vi "SP_OEE_2_test.vi"() -> ()   [LabVIEW 2017] (continued)
                      tunnel: [w10534] -> w10370
                      tunnel: [w10533] -> w10369
                      tunnel: [w10532] -> w10368
                      tunnel: [w10531] -> w10367
                      tunnel: [w10528] -> w10366
                      tunnel: [w10522] -> w10365
                      tunnel: [w10521] -> w10364
                      tunnel: [w10526] -> w10363
                      tunnel: [w10525] -> w10362
                      tunnel: [w10524] -> w10361
                      tunnel: w10374 -> [w10520]
                      tunnel: [w10520] -> w10360
                      tunnel: w10373 -> [w10517]
                      tunnel: [w10517] -> w10359
                      tunnel: [w10516] -> w10358
                      tunnel: w10372 -> [w10516]
                      tunnel: w10305 -> [w10515]
                      tunnel: [w10515] -> w10304
                      tunnel: w10299 -> [w10514]
                      tunnel: [w10514] -> w10298
                      tunnel: w10371 -> [w10559]
                      tunnel: w10370 -> [w10558]
                      tunnel: w10369 -> [w10557]
                      tunnel: w10368 -> [w10556]
                      tunnel: w10367 -> [w10555]
                      tunnel: w10366 -> [w10551]
                      tunnel: w10365 -> [w10554]
                      tunnel: w10364 -> [w10553]
                      tunnel: w10363 -> [w10550]
                      tunnel: w10362 -> [w10547]
                      tunnel: w10361 -> [w10546]
                      tunnel: [w10559] -> w10357
                      tunnel: [w10558] -> w10356
                      tunnel: [w10557] -> w10355
                      tunnel: [w10556] -> w10354
                      tunnel: [w10555] -> w10353
                      tunnel: [w10554] -> w10352
                      tunnel: [w10553] -> w10351
                      tunnel: [w10549] -> w10350
                      tunnel: [w10548] -> w10349
                      tunnel: [w10544] -> w10348
                      tunnel: [w10543] -> w10347
                      tunnel: [w10547] -> w10346
                      tunnel: [w10546] -> w10345
                      tunnel: w10360 -> [w10542]
                      tunnel: [w10542] -> w10344
                      tunnel: w10359 -> [w10539]
                      tunnel: [w10539] -> w10343
                      tunnel: [w10538] -> w10342
                      tunnel: w10358 -> [w10538]
                      tunnel: w10304 -> [w10537]
                      tunnel: [w10537] -> w10303
                      tunnel: w10298 -> [w10536]
                      tunnel: [w10536] -> w10297
                      tunnel: w10357 -> [w10585]
                      tunnel: w10356 -> [w10584]
                      tunnel: w10355 -> [w10583]
                      tunnel: w10354 -> [w10582]
                      tunnel: w10353 -> [w10581]
                      tunnel: w10352 -> [w10580]
                      tunnel: w10351 -> [w10579]
                      tunnel: w10350 -> [w10573]
                      tunnel: w10349 -> [w10575]
                      tunnel: w10348 -> [w10578]
                      tunnel: w10347 -> [w10577]
                      tunnel: w10346 -> [w10570]
                      tunnel: w10345 -> [w10571]
                      tunnel: [w10585] -> w10341
                      tunnel: [w10584] -> w10340
                      tunnel: [w10583] -> w10339
                      tunnel: [w10582] -> w10338
                      tunnel: [w10581] -> w10337
                      tunnel: [w10580] -> w10336
                      tunnel: [w10579] -> w10335
                      tunnel: [w10578] -> w10334
                      tunnel: [w10577] -> w10333
                      tunnel: [w10574] -> w10332
                      tunnel: [w10572] -> w10331
                      tunnel: [w10568] -> w10330
                      tunnel: [w10566] -> w10329
                      tunnel: w10344 -> [w10567]
                      tunnel: w10343 -> [w10563]
                      tunnel: [w10562] -> w10328
                      tunnel: w10342 -> [w10562]
                      tunnel: w10303 -> [w10561]
                      tunnel: w10297 -> [w10560]
                      tunnel: w10341 -> [w10612]
                      tunnel: w10340 -> [w10605]
                      tunnel: w10339 -> [w10596]
                      tunnel: w10338 -> [w10604]
                      tunnel: w10337 -> [w10594]
                      tunnel: w10336 -> [w10603]
                      tunnel: w10335 -> [w10592]
                      tunnel: w10334 -> [w10602]
                      tunnel: w10333 -> [w10590]
                      tunnel: w10332 -> [w10626]
                      tunnel: w10331 -> [w10625]
                      tunnel: w10330 -> [w10601]
                      tunnel: w10329 -> [w10588]
                      tunnel: [w10626] -> w10327
                      tunnel: [w10625] -> w10326
                      tunnel: [w10619] -> w10325
                      tunnel: [w10612] -> w10324
                      tunnel: [w10611] -> w10323
                      tunnel: [w10610] -> w10322
                      tunnel: [w10609] -> w10321
                      tunnel: [w10608] -> w10320
                      tunnel: [w10607] -> w10319
                      tunnel: [w10606] -> w10318
                      tunnel: [w10605] -> w10317
                      tunnel: [w10604] -> w10316
                      tunnel: [w10603] -> w10315
                      tunnel: [w10602] -> w10314
                      tunnel: [w10601] -> w10313
                      tunnel: [w10586] -> w10312
                      tunnel: w10328 -> [w10586]
                      tunnel: [w10646] -> w10288
                      tunnel: [w10632] -> w10286
                      tunnel: w10327 -> [w10633]
                      tunnel: w10326 -> [w10646]
                      tunnel: w10325 -> [w10631]
                      tunnel: w10324 -> [w10644]
                      tunnel: w10323 -> [w10642]
                      tunnel: w10322 -> [w10640]
                      tunnel: w10321 -> [w10638]
                      tunnel: w10320 -> [w10636]
                      tunnel: w10319 -> [w10634]
                      tunnel: w10318 -> [w10627]
                      tunnel: w10317 -> [w10643]
                      tunnel: w10316 -> [w10641]
                      tunnel: w10315 -> [w10639]
                      tunnel: w10314 -> [w10637]
                      tunnel: w10313 -> [w10635]
                      tunnel: w10312 -> [w10630]
                      tunnel: [w10627] -> w10296
                      frame #0 {
                        w10417 = "%Y-%m-%d" ("time format string (%c)")
                        n1887 = Decimal String To Number(string=w10404) -> (number=w10403:i32)  [unwired: 2 in, 1 out]
                        n1888 = property on="Table" class="Tbl (strict)"("Visible"=TRUE) -> ()  [unwired: 2 in, 2 out]
                        n1889 = Format Date/Time String(time format string (%c)=w10417, seconds (now)=w10409) -> (date/time string=w10418:string)  [unwired: 1 in]
                        n1890 = Format Date/Time String(time format string (%c)=w10417, seconds (now)=w10408) -> (date/time string=w10416:string)  [unwired: 1 in]
                        n1891 = Format Into String(format string="Where BREAKDOWN_DATE between '%s' and '%s' and  SHIFT_ID = '%d'  ", w10418, w10416, w10403) -> (resulting string=w10415:string)  [unwired: 2 in, 1 out]
                        n1892 = call <vilib>:"DB Tools Select Data.vi"("condition"=w10415, "error in (no error)"=w10424, "columns"=string[] ["BREAKDOWN_DATE"], "table"="STATION_1_LOG_HISTORY", "connection reference"=w10426) -> ("error out"=w10411:errorcluster, "data"=w10414:variant[][], "connection reference out"=w10425:T2)  [unwired: 1 in]
                        n1893 = property on="Table 2" class="Tbl (strict)"("Visible"=FALSE) -> ()  [unwired: 2 in, 2 out]
                        n1894 = xnode "Database Variant To Data"("database variant"=w10414, "error in (no error)"=w10411, "type"=string[][] [] ("Elements Found")) -> ("data"=w10412:string[][], "error out"=w10410:errorcluster)
                        n1895 = Index Array(array=w10412, index (col)=0 ("disabled index (col)")) -> (element=w10420:string[])  [unwired: 1 in]
                        n1896 = call "Search_1d_array_element.vi"("Count in"=string[] [] ("Elements Found"), "BD Date"=w10420, "Elements Found in"=string[] [] ("Elements Found")) -> ("Elements Found out"=w10406:string[])  [unwired: 4 in, 2 out]
                        n1897 = Build Array(w10406) -> (w10430:string[][])
                        n1898 = Transpose 2D Array(2D array=w10430) -> (transposed array=w10429:string[][])
                      }
                      frame #1 {
                        n1899 = call "Stack_holderwise_total_bd_count_&_duration_3_for_stationwise.vi"("Refnum in"=w10493, "BREAKDOWN_STK_HOLD_ID"=1, "condition"=w10480, "Form Date"=w10487, "To Date"=w10486, "error in (no error)"=w10491, "STATION_ID_CID_TRIGGER"=w10476, "Shift"=w10477) -> ("Refnum out"=w10492:T2, "Count out"=w10485:string[], "appended array"=w10482:dbl[], "error out"=w10490:errorcluster)  [unwired: 4 in]
                        n1900 = call "NUMERIC TO STRING.vi"("appended array"=w10482) -> ("Array"=w10481:string[])  [unwired: 4 in]
                        n1901 = call "Insert_empty_element_with_zero.vi"("searched date"=w10485, "fixed date"=w10483) -> ("O/P"=w10478:string[])  [unwired: 9 in]
                        n1902 = call "Insert_empty_element_with_zero.vi"("searched date"=w10481, "fixed date"=w10483) -> ("O/P"=w10484:string[])  [unwired: 9 in]
                      }
                      frame #2 {
                        n1903 = call "Stack_holderwise_total_bd_count_&_duration_3_for_stationwise.vi"("Refnum in"=w10508, "BREAKDOWN_STK_HOLD_ID"=2, "condition"=w10497, "Form Date"=w10505, "To Date"=w10504, "error in (no error)"=w10510, "STATION_ID_CID_TRIGGER"=w10494, "Shift"=w10495) -> ("Refnum out"=w10506:T2, "Count out"=w10503:string[], "appended array"=w10499:dbl[], "error out"=w10509:errorcluster)  [unwired: 4 in]
                        n1904 = call "Insert_empty_element_with_zero.vi"("searched date"=w10503, "fixed date"=w10500) -> ("O/P"=w10502:string[])  [unwired: 9 in]
                        n1905 = call "NUMERIC TO STRING.vi"("appended array"=w10499) -> ("Array"=w10498:string[])  [unwired: 4 in]
                        n1906 = call "Insert_empty_element_with_zero.vi"("searched date"=w10498, "fixed date"=w10500) -> ("O/P"=w10501:string[])  [unwired: 9 in]
                      }
                      frame #3 {
                        n1907 = call "Stack_holderwise_total_bd_count_&_duration_3_for_stationwise.vi"("Refnum in"=w10527, "BREAKDOWN_STK_HOLD_ID"=3, "condition"=w10517, "Form Date"=w10525, "To Date"=w10524, "error in (no error)"=w10529, "STATION_ID_CID_TRIGGER"=w10514, "Shift"=w10515) -> ("Refnum out"=w10526:T2, "Count out"=w10523:string[], "appended array"=w10519:dbl[], "error out"=w10528:errorcluster)  [unwired: 4 in]
                        n1908 = call "Insert_empty_element_with_zero.vi"("searched date"=w10523, "fixed date"=w10520) -> ("O/P"=w10522:string[])  [unwired: 9 in]
                        n1909 = call "NUMERIC TO STRING.vi"("appended array"=w10519) -> ("Array"=w10518:string[])  [unwired: 4 in]
                        n1910 = call "Insert_empty_element_with_zero.vi"("searched date"=w10518, "fixed date"=w10520) -> ("O/P"=w10521:string[])  [unwired: 9 in]
                      }
                      frame #4 {
                        n1911 = call "Stack_holderwise_total_bd_count_&_duration_3_for_stationwise.vi"("Refnum in"=w10550, "BREAKDOWN_STK_HOLD_ID"=4, "condition"=w10539, "Form Date"=w10547, "To Date"=w10546, "error in (no error)"=w10551, "STATION_ID_CID_TRIGGER"=w10536, "Shift"=w10537) -> ("Refnum out"=w10549:T2, "Count out"=w10545:string[], "appended array"=w10541:dbl[], "error out"=w10548:errorcluster)  [unwired: 4 in]
                        n1912 = call "Insert_empty_element_with_zero.vi"("searched date"=w10545, "fixed date"=w10542) -> ("O/P"=w10544:string[])  [unwired: 9 in]
                        n1913 = call "NUMERIC TO STRING.vi"("appended array"=w10541) -> ("Array"=w10540:string[])  [unwired: 4 in]
                        n1914 = call "Insert_empty_element_with_zero.vi"("searched date"=w10540, "fixed date"=w10542) -> ("O/P"=w10543:string[])  [unwired: 9 in]
                      }
                      frame #5 {
                        n1915 = call "Stack_holderwise_total_bd_count_&_duration_3_for_stationwise.vi"("Refnum in"=w10573, "BREAKDOWN_STK_HOLD_ID"=5, "condition"=w10563, "Form Date"=w10570, "To Date"=w10571, "error in (no error)"=w10575, "STATION_ID_CID_TRIGGER"=w10560, "Shift"=w10561) -> ("Refnum out"=w10572:T2, "Count out"=w10569:string[], "appended array"=w10565:dbl[], "error out"=w10574:errorcluster)  [unwired: 4 in]
                        n1916 = call "NUMERIC TO STRING.vi"("appended array"=w10565) -> ("Array"=w10564:string[])  [unwired: 4 in]
                        n1917 = call "Insert_empty_element_with_zero.vi"("searched date"=w10569, "fixed date"=w10567) -> ("O/P"=w10568:string[])  [unwired: 9 in]
                        n1918 = call "Insert_empty_element_with_zero.vi"("searched date"=w10564, "fixed date"=w10567) -> ("O/P"=w10566:string[])  [unwired: 9 in]
                      }
                      frame #6 {
                        n1919 = call "String to numeric.vi"("Array"=w10596) -> ("Array 2"=w10595:dbl[])  [unwired: 4 in]
                        n1920 = call "String to numeric.vi"("Array"=w10594) -> ("Array 2"=w10593:dbl[])  [unwired: 4 in]
                        n1921 = call "String to numeric.vi"("Array"=w10592) -> ("Array 2"=w10591:dbl[])  [unwired: 4 in]
                        n1922 = call "String to numeric.vi"("Array"=w10590) -> ("Array 2"=w10589:dbl[])  [unwired: 4 in]
                        n1923 = call "String to numeric.vi"("Array"=w10588) -> ("Array 2"=w10587:dbl[])  [unwired: 4 in]
                        n1924 = Decimal String To Number(string=w10601) -> (number=w10620:i32[])  [unwired: 2 in, 1 out]
                        n1925 = Decimal String To Number(string=w10602) -> (number=w10621:i32[])  [unwired: 2 in, 1 out]
                        n1926 = Decimal String To Number(string=w10603) -> (number=w10622:i32[])  [unwired: 2 in, 1 out]
                        n1927 = Decimal String To Number(string=w10604) -> (number=w10623:i32[])  [unwired: 2 in, 1 out]
                        n1928 = Decimal String To Number(string=w10605) -> (number=w10618:i32[])  [unwired: 2 in, 1 out]
                        n1929 = Compound Arithmetic op=ADD(w10595, w10593, w10591, w10589, w10587) -> (w10598:dbl[])
                        n1930 = Build Array(w10596) -> (w10617:string[][])
                        n1931 = Build Array(w10594) -> (w10616:string[][])
                        n1932 = Build Array(w10592) -> (w10615:string[][])
                        n1933 = Build Array(w10590) -> (w10614:string[][])
                        n1934 = Build Array(w10588) -> (w10613:string[][])
                        n1935 = Number To Fractional String(number=w10598, precision (6)=i16 2) -> (F-format string=w10597:string[])  [unwired: 2 in]
                        n1936 = Compound Arithmetic op=ADD(w10620, w10621, w10622, w10623, w10618) -> (w10624:i32[])
                        n1937 = Transpose 2D Array(2D array=w10617) -> (transposed array=w10611:string[][])
                        n1938 = Transpose 2D Array(2D array=w10616) -> (transposed array=w10610:string[][])
                        n1939 = Transpose 2D Array(2D array=w10615) -> (transposed array=w10609:string[][])
                        n1940 = Transpose 2D Array(2D array=w10614) -> (transposed array=w10608:string[][])
                        n1941 = Transpose 2D Array(2D array=w10613) -> (transposed array=w10607:string[][])
                        n1942 = Number To Decimal String(number=w10624) -> (decimal integer string=w10619:string[])  [unwired: 1 in]
                        n1943 = Build Array(w10597) -> (w10600:string[][])
                        n1944 = Transpose 2D Array(2D array=w10600) -> (transposed array=w10606:string[][])
                      }
                      frame #7 {
                        n1945 = Insert Into Array(array=w10644, index (col)=1 ("disabled index (col)"), new element #1=w10643, new element #2=w10642, new element #3=w10641, new element #4=w10640, new element #5=w10639, new element #6=w10638, new element #7=w10637, new element #8=w10636, new element #9=w10635, new element #10=w10634, new element #11=w10631, new element #12=w10627) -> (w10629:string[][])  [unwired: 1 in]
                        n1946 = call "flot graph for month n year.vi"("BD Date"=w10630, "error in (no error)"=w10633, "Count total"=w10631) -> ("error out"=w10632:errorcluster, "Run-Time Status"=w10628:cluster{"Array 2":timestamp[], dbl[]})  [unwired: 7 in]
                        n1947 = local write "Run-Time Status"(w10628) -> ()
                        n1948 = local write "Table"(w10629) -> ()
                      }
                    }
                    n1949 = call "OEE_PART_1.vi"("CYCLE TIME"=w10294, "ACTUAL PROD TIME"=w10295, "BREAKDOWN TOTAL TIME"=w10296) -> ("Numeric"=w10281:i32, "CAPACITY"=w10280:dbl, "ACTUAL TIME"=w10282:i32)  [unwired: 5 in, 1 out]
                    n1950 = call "OEE_PART_2_P.vi"("Refnum in"=w10288, "Shift"=w10290, "String"="ALL", "Select Station"=w10289, "Form Date"=w10293, "To Date"=w10292, "AVAILABLILITY TIME"=w10282, "CAPACITY"=w10280) -> ("Refnum out"=w10287:T2, "QUALITY"=w10285:dbl, "OEE"=w10283:dbl, "PERFORMANCE"=w10284:dbl)  [unwired: 2 in, 2 out]
                    n1951 = local write "PERFORMANCE"(w10284) -> ()
                    n1952 = local write "QUALITY"(w10285) -> ()
                    n1953 = local write "OEE"(w10283) -> ()
                    n1954 = local write "AVAILABLILITY TIME(MIN)"(w10282) -> ()
                    n1955 = local write "IDEAL CYCLE TIME"(w10281) -> ()
                    n1956 = local write "CAPACITY"(w10280) -> ()
                  }
                  frame "all" {
                  }
                }
              }
              frame "Safety" {
                n1957 = local read "Shift"() -> (w10647:string)
                n1958 = case shown="\"ALL\", Default" w10647 {
                  selector: w10647 -> [_ w11018 w11387 w11756 _]
                  tunnel: w10652 -> [w10657 w11023 w11392 w11761 _]
                  tunnel: w10651 -> [w10656 w11022 w11391 w11760 _]
                  tunnel: w10650 -> [w10655 w11021 w11390 w11759 _]
                  tunnel: w10649 -> [w10654 w11020 w11389 w11758 _]
                  tunnel: w10648 -> [w10653 w11019 w11388 w11757 _]
                  frame "ALL", Default {
                    n1959 = flat-sequence {
                      tunnel: w10657 -> [w10769]
                      tunnel: w10656 -> [w10767]
                      tunnel: [w10753] -> w10747
                      tunnel: [w10768] -> w10746
                      tunnel: w10655 -> [_]
                      tunnel: [w10772] -> w10745
                      tunnel: [w10752] -> w10744
                      tunnel: [w10751] -> w10743
                      tunnel: [w10749] -> w10742
                      tunnel: w10654 -> [w10752]
                      tunnel: w10653 -> [w10751]
                      tunnel: ["Where BREAKDOWN_DATE between '%s'and '%s' and BREAKDOWN_STK_HOLD_ID ='%d'  "] -> w10741
                      tunnel: [w10749] -> w10740
                      tunnel: w10747 -> [w10832]
                      tunnel: w10746 -> [w10834]
                      tunnel: w10745 -> [w10829]
                      tunnel: w10744 -> [w10828]
                      tunnel: w10743 -> [w10827]
                      tunnel: [w10831] -> w10739
                      tunnel: [w10833] -> w10738
                      tunnel: [w10829] -> w10737
                      tunnel: [w10819] -> w10736
                      tunnel: [w10825] -> w10735
                      tunnel: [w10828] -> w10734
                      tunnel: [w10827] -> w10733
                      tunnel: w10742 -> [w10824]
                      tunnel: [w10824] -> w10732
                      tunnel: w10741 -> [w10821]
                      tunnel: [w10821] -> w10731
                      tunnel: [w10820] -> w10730
                      tunnel: w10740 -> [w10820]
                      tunnel: w10739 -> [w10848]
                      tunnel: w10738 -> [w10846]
                      tunnel: w10737 -> [w10851]
                      tunnel: w10736 -> [w10850]
                      tunnel: w10735 -> [w10849]
                      tunnel: w10734 -> [w10844]
                      tunnel: w10733 -> [w10843]
                      tunnel: [w10851] -> w10729
                      tunnel: [w10850] -> w10728
                      tunnel: [w10849] -> w10727
                      tunnel: [w10847] -> w10726
                      tunnel: [w10841] -> w10725
                      tunnel: [w10840] -> w10724
                      tunnel: [w10845] -> w10723
                      tunnel: [w10844] -> w10722
                      tunnel: [w10843] -> w10721
                      tunnel: w10732 -> [w10839]
                      tunnel: [w10839] -> w10720
                      tunnel: w10731 -> [w10836]
                      tunnel: [w10836] -> w10719
                      tunnel: [w10835] -> w10718
                      tunnel: w10730 -> [w10835]
                      tunnel: w10729 -> [w10882]
                      tunnel: w10728 -> [w10881]
                      tunnel: w10727 -> [w10880]
                      tunnel: w10726 -> [w10877]
                      tunnel: w10725 -> [w10879]
                      tunnel: w10724 -> [w10878]
                      tunnel: w10723 -> [w10875]
                      tunnel: w10722 -> [w10873]
                      tunnel: w10721 -> [w10872]
                      tunnel: [w10882] -> w10717
                      tunnel: [w10881] -> w10716
                      tunnel: [w10880] -> w10715
                      tunnel: [w10879] -> w10714
                      tunnel: [w10878] -> w10713
                      tunnel: [w10876] -> w10712
                      tunnel: [w10870] -> w10711
                      tunnel: [w10869] -> w10710
                      tunnel: [w10874] -> w10709
                      tunnel: [w10873] -> w10708
                      tunnel: [w10872] -> w10707
                      tunnel: w10720 -> [w10868]
                      tunnel: [w10868] -> w10706
                      tunnel: w10719 -> [w10865]
                      tunnel: [w10865] -> w10705
                      tunnel: [w10864] -> w10704
                      tunnel: w10718 -> [w10864]
                      tunnel: w10717 -> [w10915]
                      tunnel: w10716 -> [w10914]
                      tunnel: w10715 -> [w10913]
                      tunnel: w10714 -> [w10912]
                      tunnel: w10713 -> [w10911]
                      tunnel: w10712 -> [w10908]
                      tunnel: w10711 -> [w10910]
                      tunnel: w10710 -> [w10909]
                      tunnel: w10709 -> [w10907]
                      tunnel: w10708 -> [w10904]
                      tunnel: w10707 -> [w10903]
                      tunnel: [w10915] -> w10703
                      tunnel: [w10914] -> w10702
                      tunnel: [w10913] -> w10701
                      tunnel: [w10912] -> w10700
                      tunnel: [w10911] -> w10699
                      tunnel: [w10910] -> w10698
                      tunnel: [w10909] -> w10697
                      tunnel: [w10906] -> w10696
                      tunnel: [w10905] -> w10695
                      tunnel: [w10901] -> w10694
                      tunnel: [w10900] -> w10693
                      tunnel: [w10904] -> w10692
                      tunnel: [w10903] -> w10691
                      tunnel: w10706 -> [w10899]
                      tunnel: [w10899] -> w10690
                      tunnel: w10705 -> [w10896]
                      tunnel: [w10896] -> w10689
                      tunnel: [w10895] -> w10688
                      tunnel: w10704 -> [w10895]
                      tunnel: w10703 -> [w10950]
                      tunnel: w10702 -> [w10949]
                      tunnel: w10701 -> [w10948]
                      tunnel: w10700 -> [w10947]
                      tunnel: w10699 -> [w10946]
                      tunnel: w10698 -> [w10945]
                      tunnel: w10697 -> [w10944]
                      tunnel: w10696 -> [w10939]
                      tunnel: w10695 -> [w10941]
                      tunnel: w10694 -> [w10943]
                      tunnel: w10693 -> [w10942]
                      tunnel: w10692 -> [w10936]
                      tunnel: w10691 -> [w10937]
                      tunnel: [w10950] -> w10687
                      tunnel: [w10949] -> w10686
                      tunnel: [w10948] -> w10685
                      tunnel: [w10947] -> w10684
                      tunnel: [w10946] -> w10683
                      tunnel: [w10945] -> w10682
                      tunnel: [w10944] -> w10681
                      tunnel: [w10943] -> w10680
                      tunnel: [w10942] -> w10679
                      tunnel: [w10940] -> w10678
                      tunnel: [w10938] -> w10677
                      tunnel: [w10934] -> w10676
                      tunnel: [w10932] -> w10675
                      tunnel: w10690 -> [w10933]
                      tunnel: w10689 -> [w10929]
                      tunnel: [w10928] -> w10674
                      tunnel: w10688 -> [w10928]
                      tunnel: w10687 -> [w10989]
                      tunnel: w10686 -> [w10982]
                      tunnel: w10685 -> [w10973]
                      tunnel: w10684 -> [w10981]
                      tunnel: w10683 -> [w10971]
                      tunnel: w10682 -> [w10980]
                      tunnel: w10681 -> [w10969]
                      tunnel: w10680 -> [w10979]
                      tunnel: w10679 -> [w10967]
                      tunnel: w10678 -> [w11003]
                      tunnel: w10677 -> [w11002]
                      tunnel: w10676 -> [w10978]
                      tunnel: w10675 -> [w10965]
                      tunnel: [w11003] -> w10673
                      tunnel: [w11002] -> w10672
                      tunnel: [w10996] -> w10671
                      tunnel: [w10989] -> w10670
                      tunnel: [w10988] -> w10669
                      tunnel: [w10987] -> w10668
                      tunnel: [w10986] -> w10667
                      tunnel: [w10985] -> w10666
                      tunnel: [w10984] -> w10665
                      tunnel: [w10983] -> w10664
                      tunnel: [w10982] -> w10663
                      tunnel: [w10981] -> w10662
                      tunnel: [w10980] -> w10661
                      tunnel: [w10979] -> w10660
                      tunnel: [w10978] -> w10659
                      tunnel: [w10963] -> w10658
                      tunnel: w10674 -> [w10963]
                      tunnel: [w11016] -> _
                      tunnel: [w11010] -> _
                      tunnel: w10673 -> [w11011]
                      tunnel: w10672 -> [w11016]
                      tunnel: w10671 -> [w11005]
                      tunnel: w10670 -> [w11014]
                      tunnel: w10669 -> [w11012]
                      tunnel: w10668 -> [_]
                      tunnel: w10667 -> [_]
                      tunnel: w10666 -> [_]
                      tunnel: w10665 -> [_]
                      tunnel: w10664 -> [w11006]
                      tunnel: w10663 -> [w11013]
                      tunnel: w10662 -> [_]
                      tunnel: w10661 -> [_]
                      tunnel: w10660 -> [_]
                      tunnel: w10659 -> [_]
                      tunnel: w10658 -> [w11009]
                      frame #0 {
                        w10760 = "%Y-%m-%d" ("time format string (%c)")
                        n1960 = property on="Table" class="Tbl (strict)"("Visible"=TRUE) -> ()  [unwired: 2 in, 2 out]
                        n1961 = Format Date/Time String(time format string (%c)=w10760, seconds (now)=w10752) -> (date/time string=w10761:string)  [unwired: 1 in]
                        n1962 = Format Date/Time String(time format string (%c)=w10760, seconds (now)=w10751) -> (date/time string=w10759:string)  [unwired: 1 in]
                        n1963 = Format Into String(format string="Where BREAKDOWN_DATE between '%s' and '%s' ", w10761, w10759) -> (resulting string=w10758:string)  [unwired: 2 in, 1 out]
                        n1964 = call <vilib>:"DB Tools Select Data.vi"("condition"=w10758, "error in (no error)"=w10767, "columns"=string[] ["BREAKDOWN_DATE"], "table"="STATION_1_LOG_HISTORY", "connection reference"=w10769) -> ("error out"=w10754:errorcluster, "data"=w10757:variant[][], "connection reference out"=w10768:T2)  [unwired: 1 in]
                        n1965 = property on="Table 2" class="Tbl (strict)"("Visible"=FALSE) -> ()  [unwired: 2 in, 2 out]
                        n1966 = xnode "Database Variant To Data"("database variant"=w10757, "error in (no error)"=w10754, "type"=string[][] [] ("Elements Found")) -> ("data"=w10755:string[][], "error out"=w10753:errorcluster)
                        n1967 = Index Array(array=w10755, index (col)=0 ("disabled index (col)")) -> (element=w10763:string[])  [unwired: 1 in]
                        n1968 = call "Search_1d_array_element.vi"("Count in"=string[] [] ("Elements Found"), "BD Date"=w10763, "Elements Found in"=string[] [] ("Elements Found")) -> ("Elements Found out"=w10749:string[])  [unwired: 4 in, 2 out]
                        n1969 = Build Array(w10749) -> (w10773:string[][])
                        n1970 = Transpose 2D Array(2D array=w10773) -> (transposed array=w10772:string[][])
                      }
                      frame #1 {
                        n1971 = call "Stack_holderwise_total_bd_count_&_duration.vi"("Refnum in"=w10834, "BREAKDOWN_STK_HOLD_ID"=1, "condition"=w10821, "Form Date"=w10828, "To Date"=w10827, "error in (no error)"=w10832) -> ("Refnum out"=w10833:T2, "Count out"=w10826:string[], "appended array"=w10823:dbl[], "error out"=w10831:errorcluster)  [unwired: 6 in]
                        n1972 = call "NUMERIC TO STRING.vi"("appended array"=w10823) -> ("Array"=w10822:string[])  [unwired: 4 in]
                        n1973 = call "Insert_empty_element_with_zero.vi"("searched date"=w10826, "fixed date"=w10824) -> ("O/P"=w10819:string[])  [unwired: 9 in]
                        n1974 = call "Insert_empty_element_with_zero.vi"("searched date"=w10822, "fixed date"=w10824) -> ("O/P"=w10825:string[])  [unwired: 9 in]
                      }
                      frame #2 {
                        n1975 = disable-structure shown="Enabled" {
                          disable-tunnel: w10848 -> [w10861 w10863]
                          disable-tunnel: [w10860 w10863] -> w10847
                          disable-tunnel: w10846 -> [w10859 w10862]
                          disable-tunnel: [w10857 w10862] -> w10845
                          disable-tunnel: w10844 -> [w10856 _]
                          disable-tunnel: w10843 -> [w10855 _]
                          disable-tunnel: [w10854 _] -> w10842
                          disable-tunnel: [w10853 _] -> w10838
                          disable-tunnel: w10836 -> [w10852 _]
                          frame Disabled {
                            n1976 = call "Stack_holderwise_total_bd_count_&_duration.vi"("Refnum in"=w10859, "BREAKDOWN_STK_HOLD_ID"=2, "condition"=w10852, "Form Date"=w10856, "To Date"=w10855, "error in (no error)"=w10861) -> ("Refnum out"=w10857:T2, "Count out"=w10854:string[], "appended array"=w10853:dbl[], "error out"=w10860:errorcluster)  [unwired: 6 in]
                          }
                          frame Enabled {
                          }
                        }
                        n1977 = call "Insert_empty_element_with_zero.vi"("searched date"=w10842, "fixed date"=w10839) -> ("O/P"=w10841:string[])  [unwired: 9 in]
                        n1978 = call "NUMERIC TO STRING.vi"("appended array"=w10838) -> ("Array"=w10837:string[])  [unwired: 4 in]
                        n1979 = call "Insert_empty_element_with_zero.vi"("searched date"=w10837, "fixed date"=w10839) -> ("O/P"=w10840:string[])  [unwired: 9 in]
                      }
                      frame #3 {
                        n1980 = disable-structure shown="Enabled" {
                          disable-tunnel: w10877 -> [w10891 w10894]
                          disable-tunnel: [w10890 w10894] -> w10876
                          disable-tunnel: w10875 -> [w10889 w10893]
                          disable-tunnel: [w10888 w10893] -> w10874
                          disable-tunnel: w10873 -> [w10887 _]
                          disable-tunnel: w10872 -> [w10886 _]
                          disable-tunnel: [w10885 _] -> w10871
                          disable-tunnel: [w10884 _] -> w10867
                          disable-tunnel: w10865 -> [w10883 _]
                          frame Disabled {
                            n1981 = call "Stack_holderwise_total_bd_count_&_duration.vi"("Refnum in"=w10889, "BREAKDOWN_STK_HOLD_ID"=3, "condition"=w10883, "Form Date"=w10887, "To Date"=w10886, "error in (no error)"=w10891) -> ("Refnum out"=w10888:T2, "Count out"=w10885:string[], "appended array"=w10884:dbl[], "error out"=w10890:errorcluster)  [unwired: 6 in]
                          }
                          frame Enabled {
                          }
                        }
                        n1982 = call "Insert_empty_element_with_zero.vi"("searched date"=w10871, "fixed date"=w10868) -> ("O/P"=w10870:string[])  [unwired: 9 in]
                        n1983 = call "NUMERIC TO STRING.vi"("appended array"=w10867) -> ("Array"=w10866:string[])  [unwired: 4 in]
                        n1984 = call "Insert_empty_element_with_zero.vi"("searched date"=w10866, "fixed date"=w10868) -> ("O/P"=w10869:string[])  [unwired: 9 in]
                      }
                      frame #4 {
                        n1985 = disable-structure shown="Enabled" {
                          disable-tunnel: w10908 -> [w10924 w10927]
                          disable-tunnel: w10907 -> [w10923 w10926]
                          disable-tunnel: [w10922 w10926] -> w10906
                          disable-tunnel: [w10921 w10927] -> w10905
                          disable-tunnel: w10904 -> [w10920 _]
                          disable-tunnel: w10903 -> [w10919 _]
                          disable-tunnel: [w10918 _] -> w10902
                          disable-tunnel: [w10917 _] -> w10898
                          disable-tunnel: w10896 -> [w10916 _]
                          frame Disabled {
                            n1986 = call "Stack_holderwise_total_bd_count_&_duration.vi"("Refnum in"=w10923, "BREAKDOWN_STK_HOLD_ID"=4, "condition"=w10916, "Form Date"=w10920, "To Date"=w10919, "error in (no error)"=w10924) -> ("Refnum out"=w10922:T2, "Count out"=w10918:string[], "appended array"=w10917:dbl[], "error out"=w10921:errorcluster)  [unwired: 6 in]
                          }
                          frame Enabled {
                          }
                        }
                        n1987 = call "Insert_empty_element_with_zero.vi"("searched date"=w10902, "fixed date"=w10899) -> ("O/P"=w10901:string[])  [unwired: 9 in]
                        n1988 = call "NUMERIC TO STRING.vi"("appended array"=w10898) -> ("Array"=w10897:string[])  [unwired: 4 in]
                        n1989 = call "Insert_empty_element_with_zero.vi"("searched date"=w10897, "fixed date"=w10899) -> ("O/P"=w10900:string[])  [unwired: 9 in]
                      }
                      frame #5 {
                        n1990 = disable-structure shown="Enabled" {
                          disable-tunnel: w10941 -> [w10959 w10962]
                          disable-tunnel: [w10958 w10962] -> w10940
                          disable-tunnel: w10939 -> [w10957 w10961]
                          disable-tunnel: [w10956 w10961] -> w10938
                          disable-tunnel: w10937 -> [w10955 _]
                          disable-tunnel: w10936 -> [w10954 _]
                          disable-tunnel: [w10953 _] -> w10935
                          disable-tunnel: [w10952 _] -> w10931
                          disable-tunnel: w10929 -> [w10951 _]
                          frame Disabled {
                            n1991 = call "Stack_holderwise_total_bd_count_&_duration.vi"("Refnum in"=w10957, "BREAKDOWN_STK_HOLD_ID"=5, "condition"=w10951, "Form Date"=w10954, "To Date"=w10955, "error in (no error)"=w10959) -> ("Refnum out"=w10956:T2, "Count out"=w10953:string[], "appended array"=w10952:dbl[], "error out"=w10958:errorcluster)  [unwired: 6 in]
                          }
                          frame Enabled {
                          }
                        }
                        n1992 = call "NUMERIC TO STRING.vi"("appended array"=w10931) -> ("Array"=w10930:string[])  [unwired: 4 in]
                        n1993 = call "Insert_empty_element_with_zero.vi"("searched date"=w10935, "fixed date"=w10933) -> ("O/P"=w10934:string[])  [unwired: 9 in]
                        n1994 = call "Insert_empty_element_with_zero.vi"("searched date"=w10930, "fixed date"=w10933) -> ("O/P"=w10932:string[])  [unwired: 9 in]
                      }
                      frame #6 {
                        n1995 = call "String to numeric.vi"("Array"=w10973) -> ("Array 2"=w10972:dbl[])  [unwired: 4 in]
                        n1996 = call "String to numeric.vi"("Array"=w10971) -> ("Array 2"=w10970:dbl[])  [unwired: 4 in]
                        n1997 = call "String to numeric.vi"("Array"=w10969) -> ("Array 2"=w10968:dbl[])  [unwired: 4 in]
                        n1998 = call "String to numeric.vi"("Array"=w10967) -> ("Array 2"=w10966:dbl[])  [unwired: 4 in]
                        n1999 = call "String to numeric.vi"("Array"=w10965) -> ("Array 2"=w10964:dbl[])  [unwired: 4 in]
                        n2000 = Decimal String To Number(string=w10978) -> (number=w10997:i32[])  [unwired: 2 in, 1 out]
                        n2001 = Decimal String To Number(string=w10979) -> (number=w10998:i32[])  [unwired: 2 in, 1 out]
                        n2002 = Decimal String To Number(string=w10980) -> (number=w10999:i32[])  [unwired: 2 in, 1 out]
                        n2003 = Decimal String To Number(string=w10981) -> (number=w11000:i32[])  [unwired: 2 in, 1 out]
                        n2004 = Decimal String To Number(string=w10982) -> (number=w10995:i32[])  [unwired: 2 in, 1 out]
                        n2005 = Compound Arithmetic op=ADD(w10972, w10970, w10968, w10966, w10964) -> (w10975:dbl[])
                        n2006 = Build Array(w10973) -> (w10994:string[][])
                        n2007 = Build Array(w10971) -> (w10993:string[][])
                        n2008 = Build Array(w10969) -> (w10992:string[][])
                        n2009 = Build Array(w10967) -> (w10991:string[][])
                        n2010 = Build Array(w10965) -> (w10990:string[][])
                        n2011 = Number To Fractional String(number=w10975, precision (6)=i16 2) -> (F-format string=w10974:string[])  [unwired: 2 in]
                        n2012 = Compound Arithmetic op=ADD(w10997, w10998, w10999, w11000, w10995) -> (w11001:i32[])
                        n2013 = Transpose 2D Array(2D array=w10994) -> (transposed array=w10988:string[][])
                        n2014 = Transpose 2D Array(2D array=w10993) -> (transposed array=w10987:string[][])
                        n2015 = Transpose 2D Array(2D array=w10992) -> (transposed array=w10986:string[][])
                        n2016 = Transpose 2D Array(2D array=w10991) -> (transposed array=w10985:string[][])
                        n2017 = Transpose 2D Array(2D array=w10990) -> (transposed array=w10984:string[][])
                        n2018 = Number To Decimal String(number=w11001) -> (decimal integer string=w10996:string[])  [unwired: 1 in]
                        n2019 = Build Array(w10974) -> (w10977:string[][])
                        n2020 = Transpose 2D Array(2D array=w10977) -> (transposed array=w10983:string[][])
                      }
                      frame #7 {
                        w11004 = string[] ["0"]
                        n2021 = Insert Into Array(array=w11014, index (col)=1 ("disabled index (col)"), new element #1=w11013, new element #2=w11012, new element #3=w11004, new element #4=w11004, new element #5=w11004, new element #6=w11004, new element #7=w11004, new element #8=w11004, new element #9=w11004, new element #10=w11004, new element #11=w11005, new element #12=w11006) -> (w11008:string[][])  [unwired: 1 in]
                        n2022 = call "flot graph for month n year.vi"("BD Date"=w11009, "error in (no error)"=w11011, "Count total"=w11005) -> ("error out"=w11010:errorcluster, "Run-Time Status"=w11007:cluster{"Array 2":timestamp[], dbl[]})  [unwired: 7 in]
                        n2023 = local write "Run-Time Status"(w11007) -> ()
                        n2024 = local write "Table"(w11008) -> ()
                      }
                    }
                  }
                  frame "1" {
                    n2025 = flat-sequence {
                      tunnel: w11023 -> [w11137]
                      tunnel: w11022 -> [w11135]
                      tunnel: [w11121] -> w11113
                      tunnel: [w11136] -> w11112
                      tunnel: w11021 -> [_]
                      tunnel: [w11140] -> w11111
                      tunnel: [w11120] -> w11110
                      tunnel: [w11119] -> w11109
                      tunnel: [w11118] -> w11108
                      tunnel: w11020 -> [w11120]
                      tunnel: w11019 -> [w11119]
                      tunnel: ["Where BREAKDOWN_DATE between '%s'and '%s' and BREAKDOWN_STK_HOLD_ID ='%d' and  SHIFT_ID = '%d' "] -> w11107
                      tunnel: [w11118] -> w11106
                      tunnel: w11018 -> [w11114]
                      tunnel: [w11114] -> w11017
                      tunnel: w11113 -> [w11201]
                      tunnel: w11112 -> [w11203]
                      tunnel: w11111 -> [w11198]
                      tunnel: w11110 -> [w11197]
                      tunnel: w11109 -> [w11196]
                      tunnel: [w11200] -> w11105
                      tunnel: [w11202] -> w11104
                      tunnel: [w11198] -> w11103
                      tunnel: [w11188] -> w11102
                      tunnel: [w11194] -> w11101
                      tunnel: [w11197] -> w11100
                      tunnel: [w11196] -> w11099
                      tunnel: w11108 -> [w11193]
                      tunnel: [w11193] -> w11098
                      tunnel: w11107 -> [w11190]
                      tunnel: [w11190] -> w11097
                      tunnel: [w11189] -> w11096
                      tunnel: w11106 -> [w11189]
                      tunnel: w11017 -> [w11187]
                      tunnel: w11105 -> [w11217]
                      tunnel: w11104 -> [w11215]
                      tunnel: w11103 -> [w11220]
                      tunnel: w11102 -> [w11219]
                      tunnel: w11101 -> [w11218]
                      tunnel: w11100 -> [w11213]
                      tunnel: w11099 -> [w11212]
                      tunnel: [w11220] -> w11095
                      tunnel: [w11219] -> w11094
                      tunnel: [w11218] -> w11093
                      tunnel: [w11216] -> w11092
                      tunnel: [w11210] -> w11091
                      tunnel: [w11209] -> w11090
                      tunnel: [w11214] -> w11089
                      tunnel: [w11213] -> w11088
                      tunnel: [w11212] -> w11087
                      tunnel: w11098 -> [w11208]
                      tunnel: [w11208] -> w11086
                      tunnel: w11097 -> [w11205]
                      tunnel: [w11205] -> w11085
                      tunnel: [w11204] -> w11084
                      tunnel: w11096 -> [w11204]
                      tunnel: w11095 -> [w11251]
                      tunnel: w11094 -> [w11250]
                      tunnel: w11093 -> [w11249]
                      tunnel: w11092 -> [w11246]
                      tunnel: w11091 -> [w11248]
                      tunnel: w11090 -> [w11247]
                      tunnel: w11089 -> [w11244]
                      tunnel: w11088 -> [w11242]
                      tunnel: w11087 -> [w11241]
                      tunnel: [w11251] -> w11083
                      tunnel: [w11250] -> w11082
                      tunnel: [w11249] -> w11081
                      tunnel: [w11248] -> w11080
                      tunnel: [w11247] -> w11079
                      tunnel: [w11245] -> w11078
                      tunnel: [w11239] -> w11077
                      tunnel: [w11238] -> w11076
                      tunnel: [w11243] -> w11075
                      tunnel: [w11242] -> w11074
                      tunnel: [w11241] -> w11073
                      tunnel: w11086 -> [w11237]
                      tunnel: [w11237] -> w11072
                      tunnel: w11085 -> [w11234]
                      tunnel: [w11234] -> w11071
                      tunnel: [w11233] -> w11070
                      tunnel: w11084 -> [w11233]
                      tunnel: w11083 -> [w11284]
                      tunnel: w11082 -> [w11283]
                      tunnel: w11081 -> [w11282]
                      tunnel: w11080 -> [w11281]
                      tunnel: w11079 -> [w11280]
                      tunnel: w11078 -> [w11277]
                      tunnel: w11077 -> [w11279]
                      tunnel: w11076 -> [w11278]
                      tunnel: w11075 -> [w11276]
                      tunnel: w11074 -> [w11273]
                      tunnel: w11073 -> [w11272]
                      tunnel: [w11284] -> w11069
                      tunnel: [w11283] -> w11068
                      tunnel: [w11282] -> w11067
                      tunnel: [w11281] -> w11066
                      tunnel: [w11280] -> w11065
                      tunnel: [w11279] -> w11064
                      tunnel: [w11278] -> w11063
                      tunnel: [w11275] -> w11062
                      tunnel: [w11274] -> w11061
                      tunnel: [w11270] -> w11060
                      tunnel: [w11269] -> w11059
                      tunnel: [w11273] -> w11058
                      tunnel: [w11272] -> w11057
                      tunnel: w11072 -> [w11268]
                      tunnel: [w11268] -> w11056
                      tunnel: w11071 -> [w11265]
                      tunnel: [w11265] -> w11055
                      tunnel: [w11264] -> w11054
                      tunnel: w11070 -> [w11264]
                      tunnel: w11069 -> [w11319]
                      tunnel: w11068 -> [w11318]
                      tunnel: w11067 -> [w11317]
                      tunnel: w11066 -> [w11316]
                      tunnel: w11065 -> [w11315]
                      tunnel: w11064 -> [w11314]
                      tunnel: w11063 -> [w11313]
                      tunnel: w11062 -> [w11308]
                      tunnel: w11061 -> [w11310]
                      tunnel: w11060 -> [w11312]
                      tunnel: w11059 -> [w11311]
                      tunnel: w11058 -> [w11305]
                      tunnel: w11057 -> [w11306]
                      tunnel: [w11319] -> w11053
                      tunnel: [w11318] -> w11052
                      tunnel: [w11317] -> w11051
                      tunnel: [w11316] -> w11050
                      tunnel: [w11315] -> w11049
                      tunnel: [w11314] -> w11048
                      tunnel: [w11313] -> w11047
                      tunnel: [w11312] -> w11046
                      tunnel: [w11311] -> w11045
                      tunnel: [w11309] -> w11044
                      tunnel: [w11307] -> w11043
                      tunnel: [w11303] -> w11042
                      tunnel: [w11301] -> w11041
                      tunnel: w11056 -> [w11302]
                      tunnel: w11055 -> [w11298]
                      tunnel: [w11297] -> w11040
                      tunnel: w11054 -> [w11297]
                      tunnel: w11053 -> [w11358]
                      tunnel: w11052 -> [w11351]
                      tunnel: w11051 -> [w11342]
                      tunnel: w11050 -> [w11350]
                      tunnel: w11049 -> [w11340]
                      tunnel: w11048 -> [w11349]
                      tunnel: w11047 -> [w11338]
                      tunnel: w11046 -> [w11348]
                      tunnel: w11045 -> [w11336]
                      tunnel: w11044 -> [w11372]
                      tunnel: w11043 -> [w11371]
                      tunnel: w11042 -> [w11347]
                      tunnel: w11041 -> [w11334]
                      tunnel: [w11372] -> w11039
                      tunnel: [w11371] -> w11038
                      tunnel: [w11365] -> w11037
                      tunnel: [w11358] -> w11036
                      tunnel: [w11357] -> w11035
                      tunnel: [w11356] -> w11034
                      tunnel: [w11355] -> w11033
                      tunnel: [w11354] -> w11032
                      tunnel: [w11353] -> w11031
                      tunnel: [w11352] -> w11030
                      tunnel: [w11351] -> w11029
                      tunnel: [w11350] -> w11028
                      tunnel: [w11349] -> w11027
                      tunnel: [w11348] -> w11026
                      tunnel: [w11347] -> w11025
                      tunnel: [w11332] -> w11024
                      tunnel: w11040 -> [w11332]
                      tunnel: [w11385] -> _
                      tunnel: [w11379] -> _
                      tunnel: w11039 -> [w11380]
                      tunnel: w11038 -> [w11385]
                      tunnel: w11037 -> [w11374]
                      tunnel: w11036 -> [w11383]
                      tunnel: w11035 -> [w11381]
                      tunnel: w11034 -> [_]
                      tunnel: w11033 -> [_]
                      tunnel: w11032 -> [_]
                      tunnel: w11031 -> [_]
                      tunnel: w11030 -> [w11375]
                      tunnel: w11029 -> [w11382]
                      tunnel: w11028 -> [_]
                      tunnel: w11027 -> [_]
                      tunnel: w11026 -> [_]
                      tunnel: w11025 -> [_]
                      tunnel: w11024 -> [w11378]
                      frame #0 {
                        w11128 = "%Y-%m-%d" ("time format string (%c)")
                        n2026 = Decimal String To Number(string=w11114) -> (number=w11115:i32)  [unwired: 2 in, 1 out]
                        n2027 = property on="Table" class="Tbl (strict)"("Visible"=TRUE) -> ()  [unwired: 2 in, 2 out]
                        n2028 = Format Date/Time String(time format string (%c)=w11128, seconds (now)=w11120) -> (date/time string=w11129:string)  [unwired: 1 in]
                        n2029 = Format Date/Time String(time format string (%c)=w11128, seconds (now)=w11119) -> (date/time string=w11127:string)  [unwired: 1 in]
                        n2030 = Format Into String(format string="Where BREAKDOWN_DATE between '%s' and '%s' and  SHIFT_ID = '%d'  ", w11129, w11127, w11115) -> (resulting string=w11126:string)  [unwired: 2 in, 1 out]
                        n2031 = call <vilib>:"DB Tools Select Data.vi"("condition"=w11126, "error in (no error)"=w11135, "columns"=string[] ["BREAKDOWN_DATE"], "table"="STATION_1_LOG_HISTORY", "connection reference"=w11137) -> ("error out"=w11122:errorcluster, "data"=w11125:variant[][], "connection reference out"=w11136:T2)  [unwired: 1 in]
                        n2032 = property on="Table 2" class="Tbl (strict)"("Visible"=FALSE) -> ()  [unwired: 2 in, 2 out]
                        n2033 = xnode "Database Variant To Data"("database variant"=w11125, "error in (no error)"=w11122, "type"=string[][] [] ("Elements Found")) -> ("data"=w11123:string[][], "error out"=w11121:errorcluster)
                        n2034 = Index Array(array=w11123, index (col)=0 ("disabled index (col)")) -> (element=w11131:string[])  [unwired: 1 in]
                        n2035 = call "Search_1d_array_element.vi"("Count in"=string[] [] ("Elements Found"), "BD Date"=w11131, "Elements Found in"=string[] [] ("Elements Found")) -> ("Elements Found out"=w11118:string[])  [unwired: 4 in, 2 out]
                        n2036 = Build Array(w11118) -> (w11141:string[][])
                        n2037 = Transpose 2D Array(2D array=w11141) -> (transposed array=w11140:string[][])
                      }
                      frame #1 {
                        n2038 = call "Stack_holderwise_total_bd_count_&_duration_2.vi"("Refnum in"=w11203, "BREAKDOWN_STK_HOLD_ID"=1, "condition"=w11190, "Form Date"=w11197, "To Date"=w11196, "error in (no error)"=w11201, "Shift"=w11187) -> ("Refnum out"=w11202:T2, "Count out"=w11195:string[], "appended array"=w11192:dbl[], "error out"=w11200:errorcluster)  [unwired: 5 in]
                        n2039 = call "NUMERIC TO STRING.vi"("appended array"=w11192) -> ("Array"=w11191:string[])  [unwired: 4 in]
                        n2040 = call "Insert_empty_element_with_zero.vi"("searched date"=w11195, "fixed date"=w11193) -> ("O/P"=w11188:string[])  [unwired: 9 in]
                        n2041 = call "Insert_empty_element_with_zero.vi"("searched date"=w11191, "fixed date"=w11193) -> ("O/P"=w11194:string[])  [unwired: 9 in]
                      }
                      frame #2 {
                        n2042 = disable-structure shown="Enabled" {
                          disable-tunnel: w11217 -> [w11230 w11232]
                          disable-tunnel: [w11229 w11232] -> w11216
                          disable-tunnel: w11215 -> [w11228 w11231]
                          disable-tunnel: [w11226 w11231] -> w11214
                          disable-tunnel: w11213 -> [w11225 _]
                          disable-tunnel: w11212 -> [w11224 _]
                          disable-tunnel: [w11223 _] -> w11211
                          disable-tunnel: [w11222 _] -> w11207
                          disable-tunnel: w11205 -> [w11221 _]
                          frame Disabled {
                            n2043 = call "Stack_holderwise_total_bd_count_&_duration.vi"("Refnum in"=w11228, "BREAKDOWN_STK_HOLD_ID"=2, "condition"=w11221, "Form Date"=w11225, "To Date"=w11224, "error in (no error)"=w11230) -> ("Refnum out"=w11226:T2, "Count out"=w11223:string[], "appended array"=w11222:dbl[], "error out"=w11229:errorcluster)  [unwired: 6 in]
                          }
                          frame Enabled {
                          }
                        }
                        n2044 = call "Insert_empty_element_with_zero.vi"("searched date"=w11211, "fixed date"=w11208) -> ("O/P"=w11210:string[])  [unwired: 9 in]
                        n2045 = call "NUMERIC TO STRING.vi"("appended array"=w11207) -> ("Array"=w11206:string[])  [unwired: 4 in]
                        n2046 = call "Insert_empty_element_with_zero.vi"("searched date"=w11206, "fixed date"=w11208) -> ("O/P"=w11209:string[])  [unwired: 9 in]
                      }
                      frame #3 {
                        n2047 = disable-structure shown="Enabled" {
                          disable-tunnel: w11246 -> [w11260 w11263]
                          disable-tunnel: [w11259 w11263] -> w11245
                          disable-tunnel: w11244 -> [w11258 w11262]
                          disable-tunnel: [w11257 w11262] -> w11243
                          disable-tunnel: w11242 -> [w11256 _]
                          disable-tunnel: w11241 -> [w11255 _]
                          disable-tunnel: [w11254 _] -> w11240
                          disable-tunnel: [w11253 _] -> w11236
                          disable-tunnel: w11234 -> [w11252 _]
                          frame Disabled {
                            n2048 = call "Stack_holderwise_total_bd_count_&_duration.vi"("Refnum in"=w11258, "BREAKDOWN_STK_HOLD_ID"=3, "condition"=w11252, "Form Date"=w11256, "To Date"=w11255, "error in (no error)"=w11260) -> ("Refnum out"=w11257:T2, "Count out"=w11254:string[], "appended array"=w11253:dbl[], "error out"=w11259:errorcluster)  [unwired: 6 in]
                          }
                          frame Enabled {
                          }
                        }
                        n2049 = call "Insert_empty_element_with_zero.vi"("searched date"=w11240, "fixed date"=w11237) -> ("O/P"=w11239:string[])  [unwired: 9 in]
                        n2050 = call "NUMERIC TO STRING.vi"("appended array"=w11236) -> ("Array"=w11235:string[])  [unwired: 4 in]
                        n2051 = call "Insert_empty_element_with_zero.vi"("searched date"=w11235, "fixed date"=w11237) -> ("O/P"=w11238:string[])  [unwired: 9 in]
                      }
                      frame #4 {
                        n2052 = disable-structure shown="Enabled" {
                          disable-tunnel: w11277 -> [w11293 w11296]
                          disable-tunnel: w11276 -> [w11292 w11295]
                          disable-tunnel: [w11291 w11295] -> w11275
                          disable-tunnel: [w11290 w11296] -> w11274
                          disable-tunnel: w11273 -> [w11289 _]
                          disable-tunnel: w11272 -> [w11288 _]
                          disable-tunnel: [w11287 _] -> w11271
                          disable-tunnel: [w11286 _] -> w11267
                          disable-tunnel: w11265 -> [w11285 _]
                          frame Disabled {
                            n2053 = call "Stack_holderwise_total_bd_count_&_duration.vi"("Refnum in"=w11292, "BREAKDOWN_STK_HOLD_ID"=4, "condition"=w11285, "Form Date"=w11289, "To Date"=w11288, "error in (no error)"=w11293) -> ("Refnum out"=w11291:T2, "Count out"=w11287:string[], "appended array"=w11286:dbl[], "error out"=w11290:errorcluster)  [unwired: 6 in]
                          }
                          frame Enabled {
                          }
                        }
                        n2054 = call "Insert_empty_element_with_zero.vi"("searched date"=w11271, "fixed date"=w11268) -> ("O/P"=w11270:string[])  [unwired: 9 in]
                        n2055 = call "NUMERIC TO STRING.vi"("appended array"=w11267) -> ("Array"=w11266:string[])  [unwired: 4 in]
                        n2056 = call "Insert_empty_element_with_zero.vi"("searched date"=w11266, "fixed date"=w11268) -> ("O/P"=w11269:string[])  [unwired: 9 in]
                      }
                      frame #5 {
                        n2057 = disable-structure shown="Enabled" {
                          disable-tunnel: w11310 -> [w11328 w11331]
                          disable-tunnel: [w11327 w11331] -> w11309
                          disable-tunnel: w11308 -> [w11326 w11330]
                          disable-tunnel: [w11325 w11330] -> w11307
                          disable-tunnel: w11306 -> [w11324 _]
                          disable-tunnel: w11305 -> [w11323 _]
                          disable-tunnel: [w11322 _] -> w11304
                          disable-tunnel: [w11321 _] -> w11300
                          disable-tunnel: w11298 -> [w11320 _]
                          frame Disabled {
                            n2058 = call "Stack_holderwise_total_bd_count_&_duration.vi"("Refnum in"=w11326, "BREAKDOWN_STK_HOLD_ID"=5, "condition"=w11320, "Form Date"=w11323, "To Date"=w11324, "error in (no error)"=w11328) -> ("Refnum out"=w11325:T2, "Count out"=w11322:string[], "appended array"=w11321:dbl[], "error out"=w11327:errorcluster)  [unwired: 6 in]
                          }
                          frame Enabled {
                          }
                        }
                        n2059 = call "NUMERIC TO STRING.vi"("appended array"=w11300) -> ("Array"=w11299:string[])  [unwired: 4 in]
                        n2060 = call "Insert_empty_element_with_zero.vi"("searched date"=w11304, "fixed date"=w11302) -> ("O/P"=w11303:string[])  [unwired: 9 in]
                        n2061 = call "Insert_empty_element_with_zero.vi"("searched date"=w11299, "fixed date"=w11302) -> ("O/P"=w11301:string[])  [unwired: 9 in]
                      }
                      frame #6 {
                        n2062 = call "String to numeric.vi"("Array"=w11342) -> ("Array 2"=w11341:dbl[])  [unwired: 4 in]
                        n2063 = call "String to numeric.vi"("Array"=w11340) -> ("Array 2"=w11339:dbl[])  [unwired: 4 in]
                        n2064 = call "String to numeric.vi"("Array"=w11338) -> ("Array 2"=w11337:dbl[])  [unwired: 4 in]
                        n2065 = call "String to numeric.vi"("Array"=w11336) -> ("Array 2"=w11335:dbl[])  [unwired: 4 in]
                        n2066 = call "String to numeric.vi"("Array"=w11334) -> ("Array 2"=w11333:dbl[])  [unwired: 4 in]
                        n2067 = Decimal String To Number(string=w11347) -> (number=w11366:i32[])  [unwired: 2 in, 1 out]
                        n2068 = Decimal String To Number(string=w11348) -> (number=w11367:i32[])  [unwired: 2 in, 1 out]
                        n2069 = Decimal String To Number(string=w11349) -> (number=w11368:i32[])  [unwired: 2 in, 1 out]
                        n2070 = Decimal String To Number(string=w11350) -> (number=w11369:i32[])  [unwired: 2 in, 1 out]
                        n2071 = Decimal String To Number(string=w11351) -> (number=w11364:i32[])  [unwired: 2 in, 1 out]
                        n2072 = Compound Arithmetic op=ADD(w11341, w11339, w11337, w11335, w11333) -> (w11344:dbl[])
                        n2073 = Build Array(w11342) -> (w11363:string[][])
                        n2074 = Build Array(w11340) -> (w11362:string[][])
                        n2075 = Build Array(w11338) -> (w11361:string[][])
                        n2076 = Build Array(w11336) -> (w11360:string[][])
                        n2077 = Build Array(w11334) -> (w11359:string[][])
                        n2078 = Number To Fractional String(number=w11344, precision (6)=i16 2) -> (F-format string=w11343:string[])  [unwired: 2 in]
                        n2079 = Compound Arithmetic op=ADD(w11366, w11367, w11368, w11369, w11364) -> (w11370:i32[])
                        n2080 = Transpose 2D Array(2D array=w11363) -> (transposed array=w11357:string[][])
                        n2081 = Transpose 2D Array(2D array=w11362) -> (transposed array=w11356:string[][])
                        n2082 = Transpose 2D Array(2D array=w11361) -> (transposed array=w11355:string[][])
                        n2083 = Transpose 2D Array(2D array=w11360) -> (transposed array=w11354:string[][])
                        n2084 = Transpose 2D Array(2D array=w11359) -> (transposed array=w11353:string[][])
                        n2085 = Number To Decimal String(number=w11370) -> (decimal integer string=w11365:string[])  [unwired: 1 in]
                        n2086 = Build Array(w11343) -> (w11346:string[][])
                        n2087 = Transpose 2D Array(2D array=w11346) -> (transposed array=w11352:string[][])
                      }
                      frame #7 {
                        w11373 = string[] [""]
                        n2088 = Insert Into Array(array=w11383, index (col)=1 ("disabled index (col)"), new element #1=w11382, new element #2=w11381, new element #3=w11373, new element #4=w11373, new element #5=w11373, new element #6=w11373, new element #7=w11373, new element #8=w11373, new element #9=w11373, new element #10=w11373, new element #11=w11374, new element #12=w11375) -> (w11377:string[][])  [unwired: 1 in]
                        n2089 = call "flot graph for month n year.vi"("BD Date"=w11378, "error in (no error)"=w11380, "Count total"=w11374) -> ("error out"=w11379:errorcluster, "Run-Time Status"=w11376:cluster{"Array 2":timestamp[], dbl[]})  [unwired: 7 in]
                        n2090 = local write "Run-Time Status"(w11376) -> ()
                        n2091 = local write "Table"(w11377) -> ()
                      }
                    }
                  }
                  frame "2" {
                    n2092 = flat-sequence {
                      tunnel: w11392 -> [w11506]
                      tunnel: w11391 -> [w11504]
                      tunnel: [w11490] -> w11482
                      tunnel: [w11505] -> w11481
                      tunnel: w11390 -> [_]
                      tunnel: [w11509] -> w11480
                      tunnel: [w11489] -> w11479
                      tunnel: [w11488] -> w11478
                      tunnel: [w11487] -> w11477
                      tunnel: w11389 -> [w11489]
                      tunnel: w11388 -> [w11488]
                      tunnel: ["Where BREAKDOWN_DATE between '%s'and '%s' and BREAKDOWN_STK_HOLD_ID ='%d' and  SHIFT_ID = '%d' "] -> w11476
                      tunnel: [w11487] -> w11475
                      tunnel: w11387 -> [w11483]
                      tunnel: [w11483] -> w11386
                      tunnel: w11482 -> [w11570]
                      tunnel: w11481 -> [w11572]
                      tunnel: w11480 -> [w11567]
                      tunnel: w11479 -> [w11566]
                      tunnel: w11478 -> [w11565]
                      tunnel: [w11569] -> w11474
                      tunnel: [w11571] -> w11473
                      tunnel: [w11567] -> w11472
                      tunnel: [w11557] -> w11471
                      tunnel: [w11563] -> w11470
                      tunnel: [w11566] -> w11469
                      tunnel: [w11565] -> w11468
                      tunnel: w11477 -> [w11562]
                      tunnel: [w11562] -> w11467
                      tunnel: w11476 -> [w11559]
                      tunnel: [w11559] -> w11466
                      tunnel: [w11558] -> w11465
                      tunnel: w11475 -> [w11558]
                      tunnel: w11386 -> [w11556]
                      tunnel: w11474 -> [w11586]
                      tunnel: w11473 -> [w11584]
                      tunnel: w11472 -> [w11589]
                      tunnel: w11471 -> [w11588]
                      tunnel: w11470 -> [w11587]
                      tunnel: w11469 -> [w11582]
                      tunnel: w11468 -> [w11581]
                      tunnel: [w11589] -> w11464
                      tunnel: [w11588] -> w11463
                      tunnel: [w11587] -> w11462
                      tunnel: [w11585] -> w11461
                      tunnel: [w11579] -> w11460
                      tunnel: [w11578] -> w11459
                      tunnel: [w11583] -> w11458
                      tunnel: [w11582] -> w11457
                      tunnel: [w11581] -> w11456
                      tunnel: w11467 -> [w11577]
                      tunnel: [w11577] -> w11455
                      tunnel: w11466 -> [w11574]
                      tunnel: [w11574] -> w11454
                      tunnel: [w11573] -> w11453
                      tunnel: w11465 -> [w11573]
                      tunnel: w11464 -> [w11620]
                      tunnel: w11463 -> [w11619]
                      tunnel: w11462 -> [w11618]
                      tunnel: w11461 -> [w11615]
                      tunnel: w11460 -> [w11617]
                      tunnel: w11459 -> [w11616]
                      tunnel: w11458 -> [w11613]
                      tunnel: w11457 -> [w11611]
                      tunnel: w11456 -> [w11610]
                      tunnel: [w11620] -> w11452
                      tunnel: [w11619] -> w11451
                      tunnel: [w11618] -> w11450
                      tunnel: [w11617] -> w11449
                      tunnel: [w11616] -> w11448
                      tunnel: [w11614] -> w11447
                      tunnel: [w11608] -> w11446
                      tunnel: [w11607] -> w11445
                      tunnel: [w11612] -> w11444
                      tunnel: [w11611] -> w11443
                      tunnel: [w11610] -> w11442
                      tunnel: w11455 -> [w11606]
                      tunnel: [w11606] -> w11441
                      tunnel: w11454 -> [w11603]
                      tunnel: [w11603] -> w11440
                      tunnel: [w11602] -> w11439
                      tunnel: w11453 -> [w11602]
                      tunnel: w11452 -> [w11653]
                      tunnel: w11451 -> [w11652]
                      tunnel: w11450 -> [w11651]
                      tunnel: w11449 -> [w11650]
                      tunnel: w11448 -> [w11649]
                      tunnel: w11447 -> [w11646]
                      tunnel: w11446 -> [w11648]
                      tunnel: w11445 -> [w11647]
                      tunnel: w11444 -> [w11645]
                      tunnel: w11443 -> [w11642]
                      tunnel: w11442 -> [w11641]
                      tunnel: [w11653] -> w11438
                      tunnel: [w11652] -> w11437
                      tunnel: [w11651] -> w11436
                      tunnel: [w11650] -> w11435
                      tunnel: [w11649] -> w11434
                      tunnel: [w11648] -> w11433
                      tunnel: [w11647] -> w11432
                      tunnel: [w11644] -> w11431
                      tunnel: [w11643] -> w11430
                      tunnel: [w11639] -> w11429
                      tunnel: [w11638] -> w11428
                      tunnel: [w11642] -> w11427
                      tunnel: [w11641] -> w11426
                      tunnel: w11441 -> [w11637]
                      tunnel: [w11637] -> w11425
                      tunnel: w11440 -> [w11634]
                      tunnel: [w11634] -> w11424
                      tunnel: [w11633] -> w11423
                      tunnel: w11439 -> [w11633]
                      tunnel: w11438 -> [w11688]
                      tunnel: w11437 -> [w11687]
                      tunnel: w11436 -> [w11686]
                      tunnel: w11435 -> [w11685]
                      tunnel: w11434 -> [w11684]
